vi "Gasringtestbetrieb.vi"(6 "Aktion":enum16{"lesen", "schreiben"}(ring), 10 "Speed":u16, 11 "Manuell":u16) -> (2 "Speed":dbl, 3 "Manuell":bool)   [LabVIEW 2020, in "Regler.lvlib"]
uses:
  Regler.lvlib
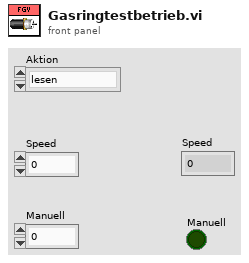
[diagram p1: front panel]
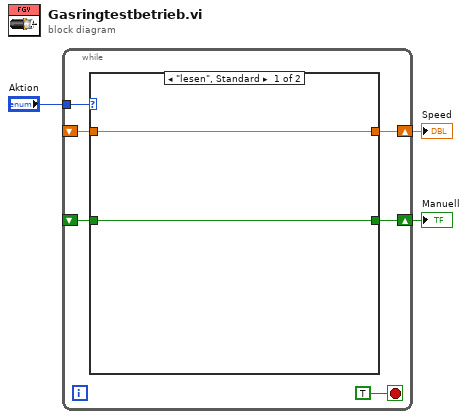
[diagram p0: block diagram]
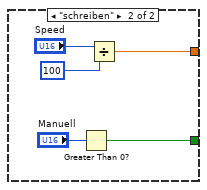
[diagram p2: hidden frame]
diagram:
  n1 = while {
    tunnel: "Aktion" -> [w8]
    shift-right: [w7] -> w2
    shift-left: _ -> [w6]
    shift-right: [w5] -> w1
    shift-left: _ -> [w4]
    stop <- TRUE stop-if-true
    n2 = case shown="\"lesen\", Standard" w8 {
      tunnel: [w11 w14] -> w7
      tunnel: w6 -> [w11 _]
      tunnel: [w10 w12] -> w5
      tunnel: w4 -> [w10 _]
      frame "lesen", Default {
      }
      frame "schreiben" {
        n3 = Greater Than 0?(x="Manuell") -> (x > 0?=w12:bool)
        n4 = Divide(x="Speed", y=u16 100) -> (x/y=w14:dbl)
      }
    }
  }
  "Speed" <- w2
  "Manuell" <- w1
